vi "Practica8.vi"() -> ()   [LabVIEW 2024]
uses:
  <vilib>/LabVIEW Interface for Arduino/Type Defs/Pin Mode.ctl
  <vilib>/LabVIEW Interface for Arduino/Type Defs/Connection Type.ctl
  <vilib>/LabVIEW Interface for Arduino/LabVIEW Interface for Arduino.lvlib
panel:
  in  "stop":bool
  in  "Boolean":bool
  in  "Pin Mode (Input)":T1
  in  "Digital I/O Pin":u8
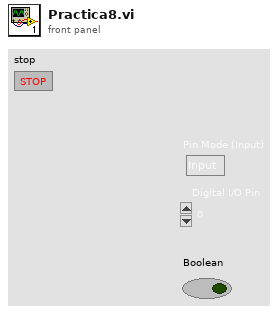
[diagram p1: front panel]
types:
  T1 = typedef "LabVIEW Interface for Arduino.lvlib/Pin Mode.ctl" = enum8{"Input", "Output"}
  T2 = typedef "LabVIEW Interface for Arduino.lvlib/Connection Type.ctl" = enum8{"USB / Serial", "XBEE", "BlueSmirf (Bluetooth)"}
  T3 = typedef "LabVIEW Interface for Arduino.lvlib/Arduino Resource.ctl" = cluster{"VISA resource":refnum<visa-resource-name>, "Board Type":T4, "Connection Type":enum8{"USB / Serial"}, "Bytes Per Packet (15)":u8}
  T4 = typedef "LabVIEW Interface for Arduino.lvlib/Board Type.ctl" = enum16{"Uno", "Dimuelanove w/Atmega 328", "Mega 2560"}
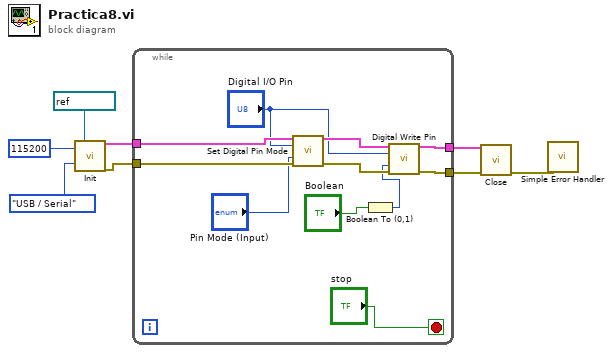
[diagram p0: block diagram]
diagram:
  n1 = call <vilib>:"Init.vi"("VISA resource"=refnum<visa-resource-name> "COM8", "Baud Rate (115200)"=u32 115200, "Connection Type (USB/Serial)"=Connection_Type."USB / Serial") -> ("Arduino Resource"=w8:T3, "error out"=w7:errorcluster)  [unwired: 15 in]
  n2 = while {
    tunnel: w8 -> [w16]
    tunnel: w7 -> [w19]
    tunnel: [w15] -> w6
    tunnel: [w14] -> w5
    stop <- "stop" stop-if-true
    n3 = call <vilib>:"Set Digital Pin Mode.vi"("Arduino Resource"=w16, "Digital I/O Pin"="Digital I/O Pin", "Pin Mode (Input)"="Pin Mode (Input)", "error in"=w19) -> ("Arduino Resource"=w18:T3, "error out"=w17:errorcluster)  [unwired: 10 in]
    n4 = Boolean To (0,1)(Boolean="Boolean") -> (0, 1=w11:i16)
    n5 = call <vilib>:"Digital Write Pin.vi"("Arduino Resource"=w18, "Digital I/O Pin (0)"="Digital I/O Pin", "Value (0)"=w11, "error in"=w17) -> ("Arduino Resource"=w15:T3, "error out"=w14:errorcluster)  [unwired: 10 in]
  }
  n6 = call <vilib>:"Close.vi"("Arduino Resource"=w6, "error in"=w5) -> ("error out"=w4:errorcluster)  [unwired: 13 in]
  n7 = call <vilib>:"Simple Error Handler.vi"("error in (no error)"=w4) -> ()  [unwired: 4 in, 5 out]
